vi "Save_dialogue_number.vi"() -> (2 "Что делаем? Номер образца? 2":string)   [LabVIEW 2013]
panel:
  in  "Что делаем? Номер образца?":string
  out "stop 2":bool
  out "OK Button 2":bool
  in  "stop":bool
  in  "OK Button":bool
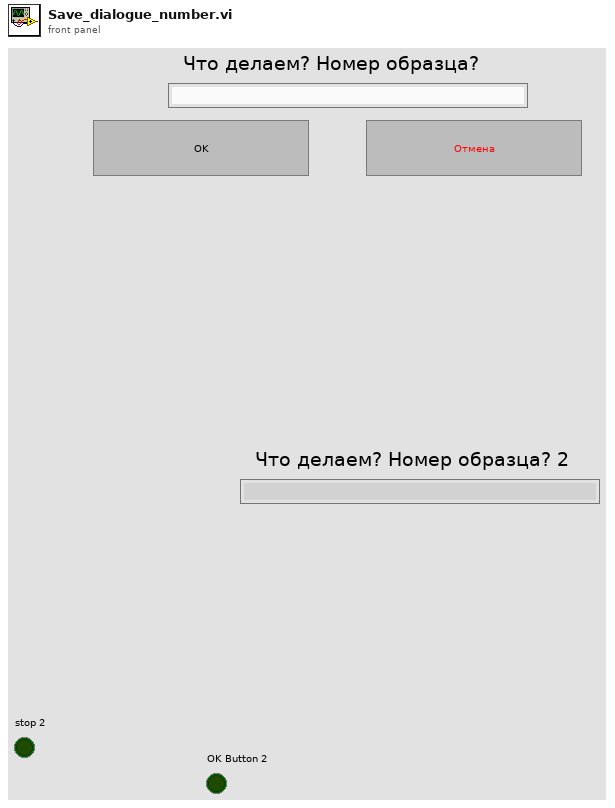
[diagram p1: front panel]
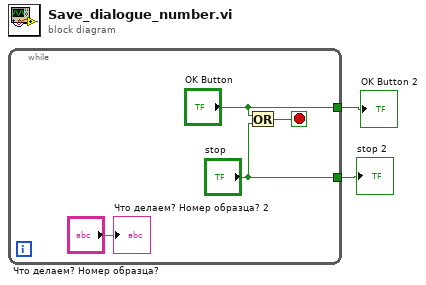
[diagram p0: block diagram]
diagram:
  n1 = while {
    tunnel: ["OK Button"] -> w2
    tunnel: ["stop"] -> w1
    stop <- w6 stop-if-true
    n2 = Or(x="OK Button", y="stop") -> (x .or. y?=w6:bool)
    "Что делаем? Номер образца? 2" <- "Что делаем? Номер образца?"
  }
  "OK Button 2" <- w2
  "stop 2" <- w1
